vi "simulate hybrid DNA and eWLC fit.vi"() -> ()   [LabVIEW 2014]
uses:
  <vilib>/gmath/NumericalOptimization/Nonlinear Curve Fit LM formula string.vi
  <vilib>/gmath/NI_Gmath.lvlib
panel:
  in  "Enum":enum16{"WLC", "modified WLC", "eWLC"}(ring)=enum."eWLC"
  out "best fit parameters for eWLC 2":dbl[](array[numeric])
  in  "initial parameters for eWLC (Lc,Lp,K)":dbl[](array[numeric])=[1000.0, 1200.0]
  out "best fit parameters for eWLC":dbl[](array[numeric])
  out "best fit parameters for WLC":dbl[](array[numeric])
  in  "initial parameters for eWLC (Lp,Lc,K)":dbl[](array[numeric])=[45.0, 1200.0, 1200.0]
  in  "initial parameters for WLC (Lp,Lc)":dbl[](array[numeric])=[45.0, 1800.0]
  in  "ssDNA Length (nt)":dbl=33.0
  in  "dsDNA Length (bp)":dbl=3371.0
  out "expected contour length for ssDNA (nm) 2":dbl
  out "expected contour length for dsDNA (nm)":dbl
  in  "Tab Control":enum32{"Page 3", "Page 1"}(tab)
  out "Raw-XY Graph 2":cluster{dbl[], dbl[]}(graph)
  out "Fit-XY Graph":cluster{dbl[], "best nonlinear fit":dbl[]}[](graph)
  out "Force Array (pN)":dbl[](array[numeric])
  in  "End Force (pN)":dbl=50.0
  in  "dF (pN)":dbl=0.1
  in  "Start Force (pN)":dbl=6.0
  # "Lp=0.37 nm and Lc=0.28 nm for PEG"
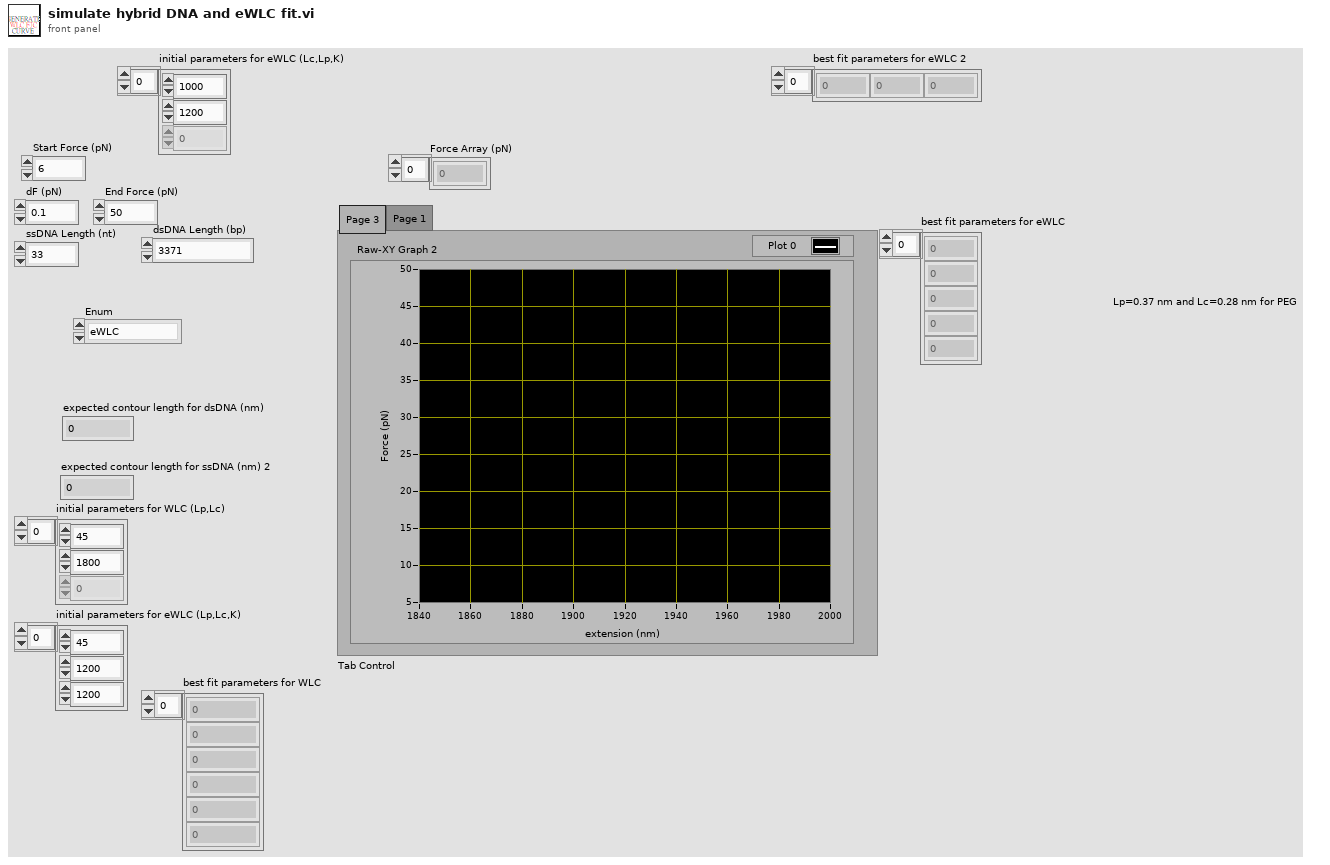
[diagram p1: front panel]
types:
  T1 = cluster{"model":string, "Parameters":string[], "x":string}
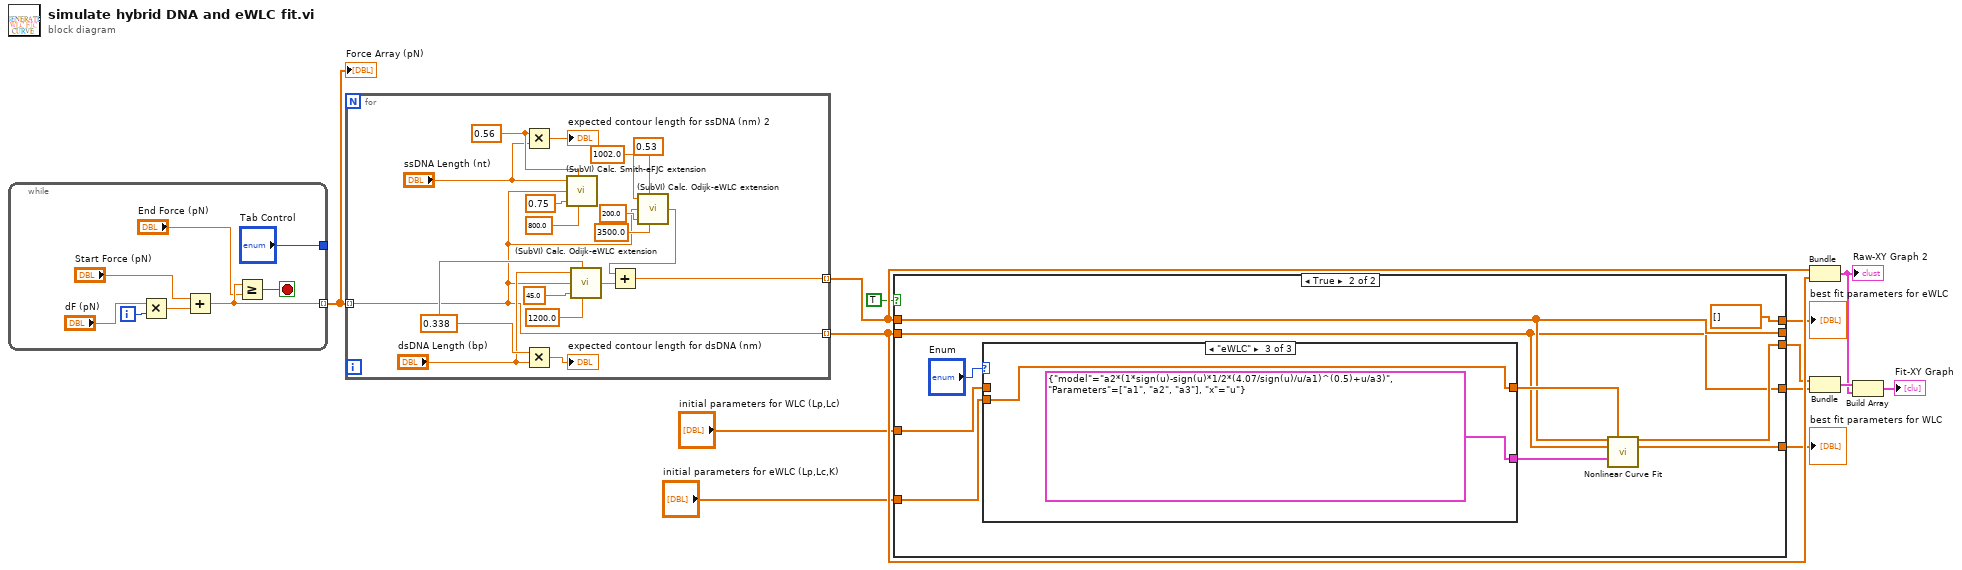
[diagram p0: block diagram]
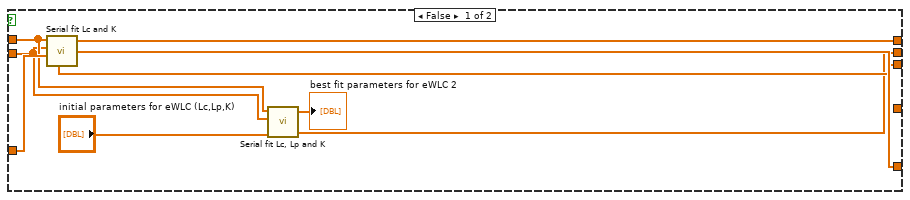
[diagram p2: hidden frame]
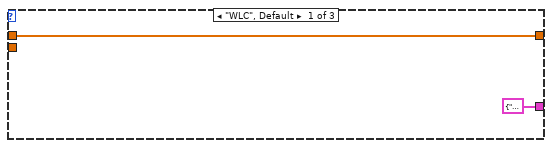
[diagram p3: hidden frame]
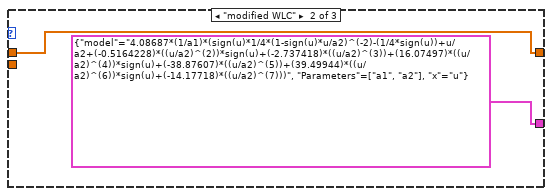
[diagram p4: hidden frame]
diagram:
  n1 = while {
    tunnel: [w17] -> w13 mode=indexing
    tunnel: ["Tab Control"] -> _
    i -> [w20]
    stop <- w15 stop-if-true
    n2 = Multiply(x="dF (pN)", y=w20) -> (x*y=w19:dbl)
    n3 = Add(x="Start Force (pN)", y=w19) -> (x+y=w17:dbl)
    n4 = Greater Or Equal?(x=w17, y="End Force (pN)") -> (x >= y?=w15:bool)
  }
  "Force Array (pN)" <- w13
  n5 = for {
    tunnel: w13 -> [w23] mode=indexing
    tunnel: [w38] -> w11 mode=indexing
    tunnel: [w23] -> w12 mode=indexing
    w37 = 0.338 ("nm/bp")
    w35 = 0.56 ("nm/nt")
    n6 = Multiply(x=w35, y="ssDNA Length (nt)") -> (x*y=→"expected contour length for ssDNA (nm) 2":dbl)
    n7 = Multiply(x=w37, y="dsDNA Length (bp)") -> (x*y=→"expected contour length for dsDNA (nm)":dbl)
    n8 = call "(SubVI) Calc. Smith-eFJC extension.vi"("ssDNA Length (nt)"="ssDNA Length (nt)", "nm/nt"=w35, "Force (pN)"=w23, "Persistence length (nm)"=0.75, "Elastic modulus (pN)"=800.0) -> ()  [unwired: 2 in, 1 out]
    n9 = call "(SubVI) Calc. Odijk-eWLC extension.vi"("dsDNA Length (bp)"="dsDNA Length (bp)", "nm/bp"=w37, "Force (pN)"=w23, "Persistence length (nm)"=45.0, "Elastic modulus (pN)"=1200.0) -> ("Extension (nm)"=w39:dbl)  [unwired: 2 in]
    n10 = call "(SubVI) Calc. Odijk-eWLC extension.vi"("dsDNA Length (bp)"=1002.0, "nm/bp"=0.53, "Force (pN)"=w23, "Persistence length (nm)"=200.0, "Elastic modulus (pN)"=3500.0) -> ("Extension (nm)"=w22:dbl)  [unwired: 2 in]
    n11 = Add(x=w22, y=w39) -> (x+y=w38:dbl)
  }
  n12 = case shown="True" TRUE {
    tunnel: w12 -> [w43 w49]
    tunnel: w11 -> [w44 w50]
    tunnel: [w40 w50] -> _
    tunnel: "initial parameters for WLC (Lp,Lc)" -> [w48 w53]
    tunnel: "initial parameters for eWLC (Lp,Lc,K)" -> [_ w51]
    tunnel: [w47 w58] -> w5
    tunnel: [w46 dbl[] [] ("best fit parameters for eWLC")] -> w4
    tunnel: [w45 w56] -> w2
    tunnel: [_ w49] -> w1
    frame False {
      n13 = call "Serial fit Lc and K.vi"("Extension (nm)"=w44, "Force (pN)"=w43, "initial parameters for WLC (Lp,Lc)"=w48) -> ("Cut-Force (pN)"=w45:dbl[], "best fit parameters for eWLC (Lp,Lc,K)"=w46:dbl[], "best fit parameters for WLC"=w47:dbl[])  [unwired: 1 in, 2 out]
      n14 = call "Serial fit Lc, Lp and K.vi"("Extension (nm)"=w44, "Force (pN)"=w43, "initial parameters for eWLC (Lc,Lp,K)"="initial parameters for eWLC (Lc,Lp,K)") -> ("best fit parameters for eWLC"=→"best fit parameters for eWLC 2":dbl[], "best nonlinear fit for eWLC"=w40:dbl[])  [unwired: 3 in, 1 out]
    }
    frame True {
      n15 = case shown="\"eWLC\"" "Enum" {
        tunnel: [T1 {"model"="4.08687*(1/a1)*(sign(u)*1/4*(1-sign(u)*u/a2)^(-2)-(1/4*sign(u))+u/a2)", "Parameters"=["a1", "a2"], "x"="u"} ("model description") T1 {"model"="4.08687*(1/a1)*(sign(u)*1/4*(1-sign(u)*u/a2)^(-2)-(1/4*sign(u))+u/a2+(-0.5164228)*((u/a2)^(2))*sign(u)+(-2.737418)*((u/a2)^(3))+(16.07497)*((u/a2)^(4))*sign(u)+(-38.87607)*((u/a2)^(5))+(39.49944)*((u/a2)^(6))*sign(u)+(-14.17718)*((u/a2)^(7)))", "Parameters"=["a1", "a2"], "x"="u"} ("model description") T1 {"model"="a2*(1*sign(u)-sign(u)*1/2*(4.07/sign(u)/u/a1)^(0.5)+u/a3)", "Parameters"=["a1", "a2", "a3"], "x"="u"} ("model description")] -> w55
        tunnel: w53 -> [w59 w61 _]
        tunnel: [w59 w61 w63] -> w52
        tunnel: w51 -> [_ _ w63]
        frame "WLC", Default {
        }
        frame "modified WLC" {
        }
        frame "eWLC" {
        }
      }
      n16 = call-poly <vilib>:"Nonlinear Curve Fit.vi"("Y"=w50, "initial parameters"=w52, "X"=w49, "model description"=w55) -> ("best nonlinear fit"=w56:dbl[], "best fit parameters"=w58:dbl[])  [unwired: 3 in, 7 out]
    }
  }
  "best fit parameters for WLC" <- w5
  "best fit parameters for eWLC" <- w4
  n17 = Bundle(w11, w12) -> (w8:cluster{dbl[], dbl[]})  [unwired: 1 in]
  "Raw-XY Graph 2" <- w8
  n18 = Bundle("best nonlinear fit"=w2, w1) -> (w10:cluster{"best nonlinear fit":dbl[], dbl[]})  [unwired: 1 in]
  n19 = Build Array(w10, w8) -> (→"Fit-XY Graph":cluster{"best nonlinear fit":dbl[], dbl[]}[])
